vi "GUI.vi"() -> ()   [LabVIEW 2014]
uses:
  sourceTypeDef.ctl
  <vilib>/express/express analysis/Spectral/Block/exnSpectralBlock spectral measurements RMS poly.vi
  <vilib>/express/express analysis/Spectral/Block/exnSpectralBlock spectral measurements RMS DDT.vi
  <vilib>/express/express analysis/Spectral/XNode/ExpressSpectralMeasurementsBlockNode.xnode
panel:
  in  "MainTabs":enum32{"Input", "Filter", "Output"}(tab)
  out "Frequency domain":dynamicdata(graph) caption="Sine"
  in  "sourceIN":enum32{"Sound file", "Simulate"}(tab)
  in  "StopFile":bool
  in  "PlayInput":bool
  in  "Input file":path
  in  "Source 3":T1
  in  "Source 2":T1
  in  "Operation":enum16{"Add", "Multiply"}(ring)
  in  "Source 1":T1
  out "Time domain":dynamicdata(graph) caption="Sine"
  in  "Filter type":enum16{""}(ring)
  out "Frequency response":dynamicdata(graph) caption="Sine"
  in  "Save to file":bool
  in  "Stop":bool
  in  "Play":bool
  out "Output - Time domain":dynamicdata(graph) caption="Sine"
  out "Output - Frequency domain":dynamicdata(graph) caption="Sine"
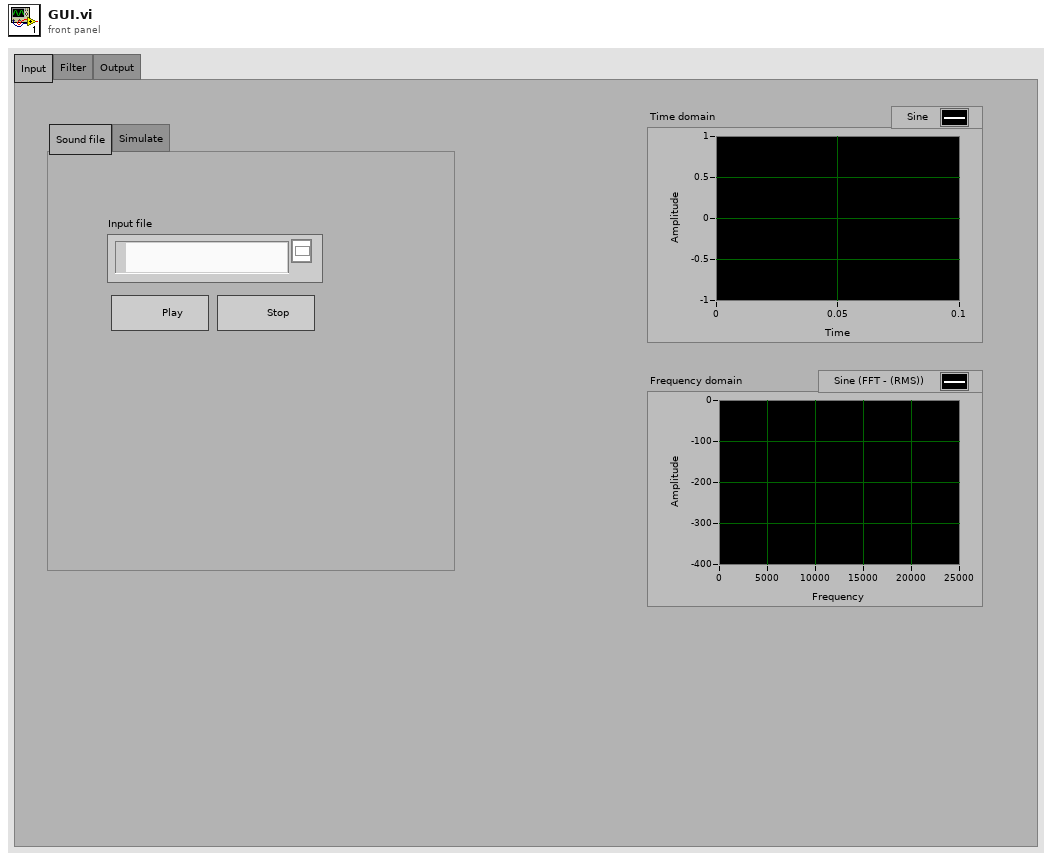
[diagram p1: front panel]
types:
  T1 = typedef "sourceTypeDef.ctl" = cluster{"Type":enum16{"Sine", "Square", "Triangle", "Noise"}, "Frequency (Hz)":dbl, "Phase (deg)":dbl}
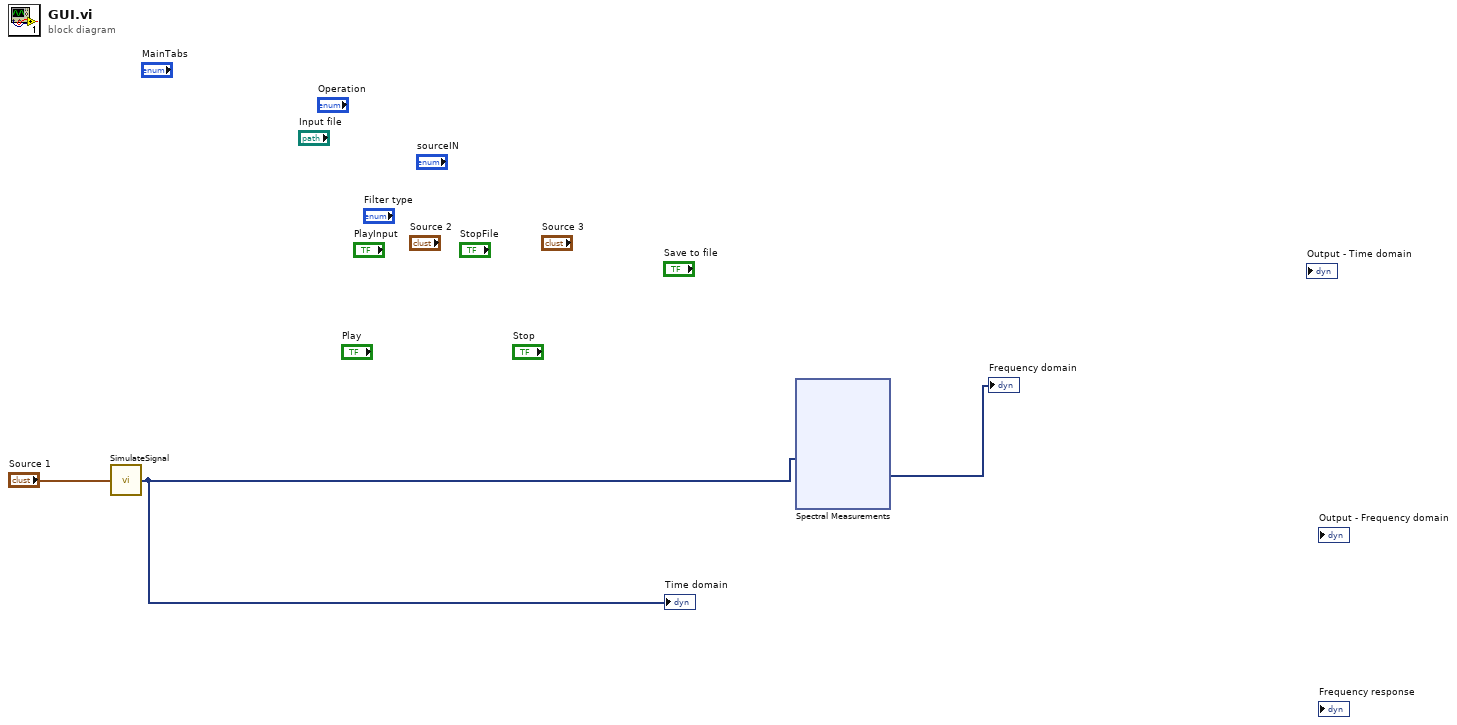
[diagram p0: block diagram]
diagram:
  n1 = call "SimulateSignal.vi"("Source"="Source 1") -> ("Waveform Graph"=w1:dynamicdata)
  "Time domain" <- w1
  n2 = xnode "Spectral Measurements"("Signals"=w1) -> ("FFT - (RMS)"=→"Frequency domain":dynamicdata)  [unwired: 1 in, 2 out]
